vi "ByRef Write.vi"   [LabVIEW 2020]
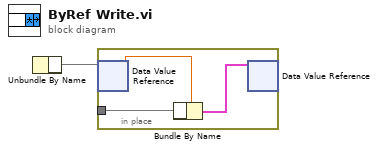
[diagram p0: block diagram]
diagram:
  n1 = Unbundle By Name() -> (w1)  [unwired: 1 in]
  n2 = in-place {
    in-place-border: _ -> [w2]
    n3 = in-place-dvr #1(w1) -> (w4:dbl)  [unwired: 1 out]
    n4 = Bundle By Name(cluster=w4, w2) -> (w3:cluster{})
    n5 = in-place-dvr #1(w3) -> ()  [unwired: 2 out]
  }
